vi "TRITON_READ_P6_COMMAND.vi"() -> (0 "Pressures Command String":string="p.pressures()")   [LabVIEW 2009]
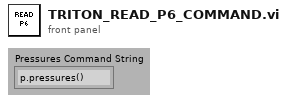
[diagram p1: front panel]
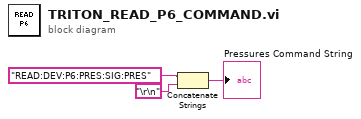
[diagram p0: block diagram]
diagram:
  n1 = Concatenate Strings("READ:DEV:P6:PRES:SIG:PRES", "\r\n") -> (→"Pressures Command String":string)
